vi "IT-M3400 New Output DC Volts.vi"() -> ()   [LabVIEW 2020]
doc: "This example shows how to configure the instrument's output voltage level, over current protection, and over voltage protection. The actual voltage level and actual current level are returned as well as whether over voltage protection (OVP) or over current protection (OCP) has been tripped."
uses:
  <instrlib>/IT-M3400/IT-M3400.lvlib
panel:
  in  "OCP Delay(s)":dbl
  in  "OVP Delay(s)":dbl
  in  "Enable OCP":bool
  in  "Current limit (A)":dbl
  in  "Channel":i32(ring)=1 items=["Channel 1"=1, "Channel 2"=2, "Channel 3"=3, "Channel 4"=4, "Channel 5"=5, "Channel 6"=6, "Channel 7"=7, "Channel 8"=8, "Channel 8"=9, "Channel 10"=10, "Channel 11"=11, "Channel 12"=12, "Channel 13"=13, "Channel 14"=14, "Channel 15"=15, "Channel 16"=16]
  in  "Enable OVP":bool
  in  "Serial Configuration":T1={"Baud Rate"=9600, "Parity"=0, "Data Bits"=8, "Stop Bits"=10, "Flow Control"=0} {"Flow Control" items=["None", "XON/XOFF", "RTS/CTS", "XON/XOFF & RTS/CTS", "DTR/DSR", "XON/XOFF & DTR/DSR"]; "Stop Bits" items=["1.0"=10, "1.5"=15, "2.0"=20]; "Data Bits" items=["7"=7, "8"=8]; "Parity" items=["None", "Odd", "Even", "Mark", "Space"]; "Baud Rate" items=["300"=300, "600"=600, "1200"=1200, "2400"=2400, "4800"=4800, "9600"=9600, "19200"=19200]}
  in  "Stop Output":bool
  in  "OVP Level(V)":dbl format="%.2f"
  out "Read Current(A)":dbl format="%.4f"
  out "Read Voltage(V)":dbl format="%.4f"
  in  "Voltage Level (V)":dbl format="%.2f"
  in  "OCP Level(A)":dbl format="%.2f"
  in  "VISA resource name":refnum<visa-resource-name>
  # "Source Output"
  # "Over Voltage Protection"
  # "Over Current Protection"
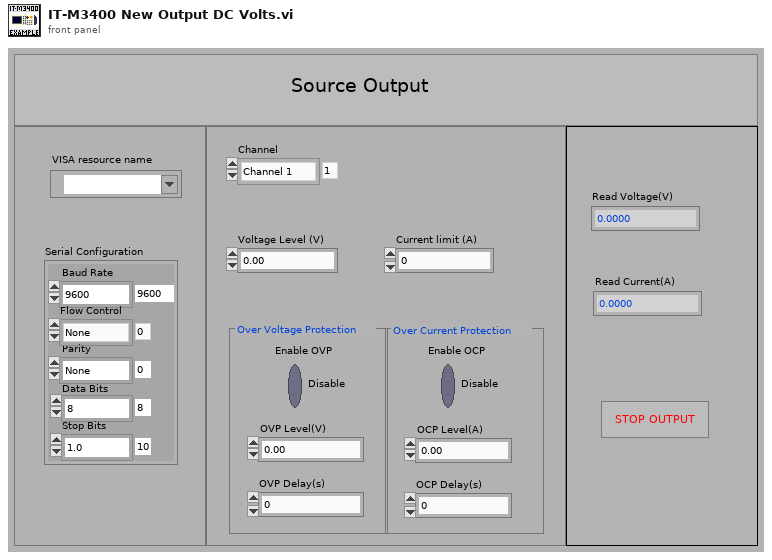
[diagram p1: front panel]
types:
  T1 = cluster{"Baud Rate":u32, "Parity":u16, "Data Bits":u16, "Stop Bits":u16, "Flow Control":u16}
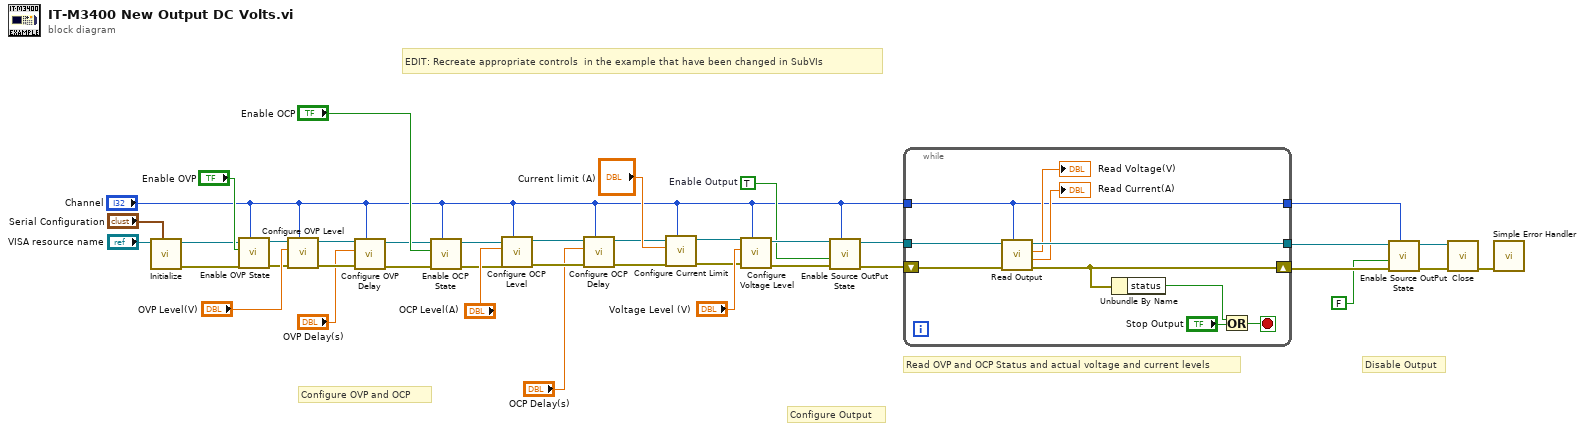
[diagram p0: block diagram]
diagram:
  w26 = TRUE  # Enable Output
  # "EDIT: Recreate appropriate controls  in the example that have been changed in SubVIs"
  # "Disable Output"
  # "Read OVP and OCP Status and actual voltage and current levels"
  # "Configure Output"
  # "Configure OVP and OCP"
  n1 = call <instrlib>:"Initialize.vi"("Serial Configuration"="Serial Configuration", "VISA resource name"="VISA resource name") -> ("error out"=w33:errorcluster, "VISA resource name out"=w34:refnum<visa-resource-name>)  [unwired: 8 in]
  n2 = call <instrlib>:"Enable OVP State.vi"("Channel"="Channel", "error in"=w33, "State"="Enable OVP", "VISA resource name"=w34) -> ("error out"=w31:errorcluster, "VISA resource name out"=w32:refnum<visa-resource-name>)  [unwired: 6 in]
  n3 = call <instrlib>:"Configure OVP Level.vi"("Channel"="Channel", "error in"=w31, "OVP Level(V)"="OVP Level(V)", "VISA resource name"=w32) -> ("error out"=w10:errorcluster, "VISA resource name out"=w11:refnum<visa-resource-name>)  [unwired: 6 in]
  n4 = call <instrlib>:"Configure OVP Delay.vi"("Channel"="Channel", "error in"=w10, "OVP Delay(S)"="OVP Delay(s)", "VISA resource name"=w11) -> ("error out"=w8:errorcluster, "VISA resource name out"=w9:refnum<visa-resource-name>)  [unwired: 6 in]
  n5 = call <instrlib>:"Enable OCP State.vi"("Channel"="Channel", "error in"=w8, "State"="Enable OCP", "VISA resource name"=w9) -> ("error out"=w15:errorcluster, "VISA resource name out"=w16:refnum<visa-resource-name>)  [unwired: 6 in]
  n6 = call <instrlib>:"Configure OCP Level.vi"("Channel"="Channel", "error in"=w15, "OCP Level(A)"="OCP Level(A)", "VISA resource name"=w16) -> ("error out"=w5:errorcluster, "VISA resource name out"=w6:refnum<visa-resource-name>)  [unwired: 6 in]
  n7 = call <instrlib>:"Configure OCP Delay.vi"("Channel"="Channel", "error in"=w5, "OCP Delay(S)"="OCP Delay(s)", "VISA resource name"=w6) -> ("error out"=w3:errorcluster, "VISA resource name out"=w4:refnum<visa-resource-name>)  [unwired: 6 in]
  n8 = call <instrlib>:"Configure Current Limit.vi"("Channel"="Channel", "error in"=w3, "Current(A)"="Current limit (A)", "VISA resource name"=w4) -> ("error out"=w12:errorcluster, "VISA resource name out"=w13:refnum<visa-resource-name>)  [unwired: 6 in]
  n9 = call <instrlib>:"Configure Voltage Level.vi"("Channel"="Channel", "error in"=w12, "Voltage(V)"="Voltage Level (V)", "VISA resource name"=w13) -> ("error out"=w27:errorcluster, "VISA resource name out"=w28:refnum<visa-resource-name>)  [unwired: 6 in]
  n10 = call <instrlib>:"Enable Source OutPut State.vi"("Channel"="Channel", "error in"=w27, "State"=w26, "VISA resource name"=w28) -> ("error out"=w24:errorcluster, "VISA resource name out"=w25:refnum<visa-resource-name>)  [unwired: 6 in]
  n11 = while {
    tunnel: w25 -> [w48]
    tunnel: [w49] -> w21
    tunnel: "Channel" -> [w40]
    tunnel: [w40] -> w19
    shift-right: [w42] -> w20
    shift-left: w24 -> [w47]
    stop <- w44 stop-if-true
    n12 = call <instrlib>:"Read Output.vi"("Channel"=w40, "error in"=w47, "VISA resource name"=w48) -> ("error out"=w42:errorcluster, "Read Current(A)"=→"Read Current(A)":dbl, "Read Voltage(V)"=→"Read Voltage(V)":dbl, "VISA resource name out"=w49:refnum<visa-resource-name>)  [unwired: 5 in]
    n13 = Unbundle By Name(w42) -> ("status"=w41:bool)
    n14 = Or(x=w41, y="Stop Output") -> (x .or. y?=w44:bool)
  }
  n15 = call <instrlib>:"Enable Source OutPut State.vi"("Channel"=w19, "error in"=w20, "State"=FALSE, "VISA resource name"=w21) -> ("error out"=w22:errorcluster, "VISA resource name out"=w23:refnum<visa-resource-name>)  [unwired: 6 in]
  n16 = call <instrlib>:"Close.vi"("error in"=w22, "VISA resource name"=w23) -> ("error out"=w38:errorcluster)  [unwired: 9 in]
  n17 = call <vilib>:"Simple Error Handler.vi"("error in (no error)"=w38) -> ()  [unwired: 4 in, 5 out]
